vi "current_to_dp.vi"(0 "Current [A]":dynamicdata(graph)) -> (1 "dP [Pa]":dbl, 2 "dP Array [Pa]":dbl[](array[numeric]))   [LabVIEW 2017]
uses:
  <vilib>/express/express arith-compare/Formula/XNode/ExpressFormulaBlockNode.xnode
  <vilib>/express/express shared/transition.llb/Dynamic To Waveform Array.vi
  <vilib>/express/express arith-compare/Formula/Block/exnFormulaBlock how many pts in the wave.vi
  <vilib>/express/express shared/ex_Modify Signal Name.vi
  <vilib>/express/express shared/transition.llb/Waveform Array To Dynamic.vi
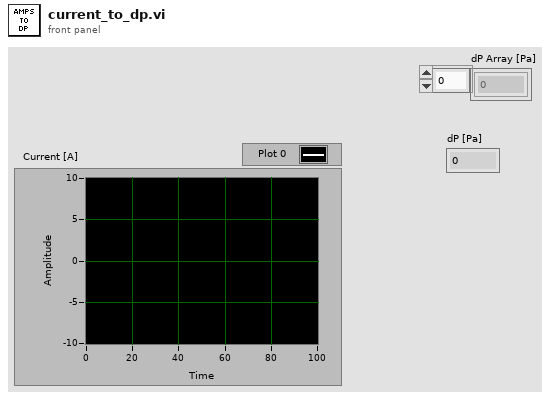
[diagram p1: front panel]
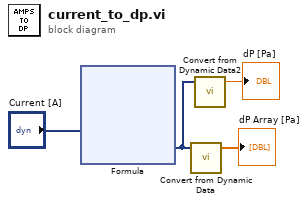
[diagram p0: block diagram]
diagram:
  n1 = xnode "Formula"("I"="Current [A]") -> ("Result"=w1:dynamicdata)  [unwired: 1 in, 1 out]
  n2 = call "Convert from Dynamic Data"("Dynamic Data Type"=w1) -> ("Array"=→"dP Array [Pa]":dbl[])  [unwired: 3 in]
  n3 = call "Convert from Dynamic Data2"("Dynamic Data Type"=w1) -> ("Scalar"=→"dP [Pa]":dbl)  [unwired: 3 in]
